vi "Find Largest Networks.vi"(8 "error in (no error)":errorcluster, 11 "Proto in":refnum<class "NetAn.lvclass">) -> (0 "error out":errorcluster, 2 "set":set{string}(c389), 3 "Proto out":refnum<class "NetAn.lvclass">)   [LabVIEW 2020, in "NetAn.lvclass"]
uses:
  NetAn.lvclass
  NetAn.lvclass/NetAn.ctl
panel:
  out "Numeric":i32
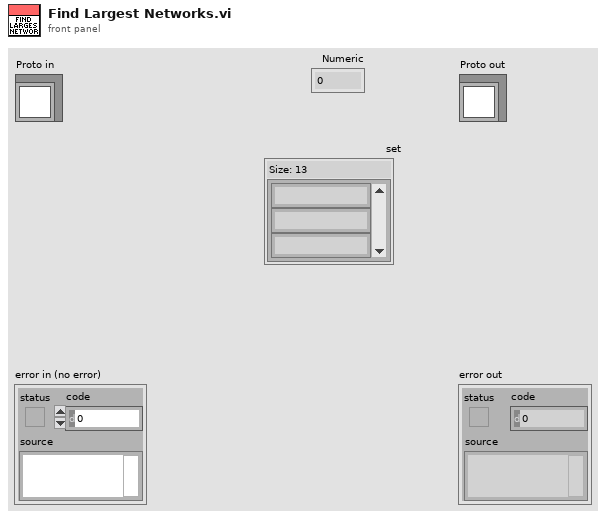
[diagram p1: front panel]
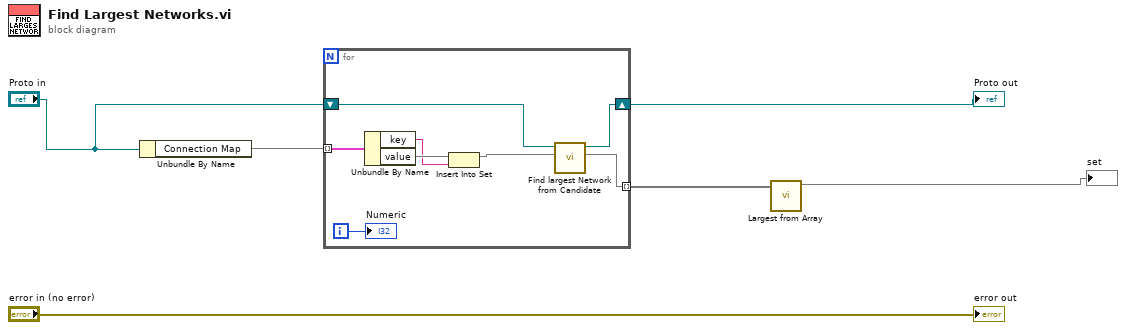
[diagram p0: block diagram]
diagram:
  n1 = Unbundle By Name("Proto in") -> ("Connection Map"=w5:map{string, set{string}})
  n2 = for {
    tunnel: w5 -> [w14] mode=indexing
    shift-right: [w8] -> w3
    shift-left: "Proto in" -> [w11]
    tunnel: [w9] -> w2 mode=indexing
    i -> [w7]
    n3 = Unbundle By Name(w14) -> ("key"=w12:string, "value"=w13:set{string})
    n4 = Insert Into Set(10:w12, 11:w13) -> (3:w10:set{string})  [unwired: 1 out]
    n5 = call "Find largest Network from Candidate.vi"("Candidate Network"=w10, "NetAn in"=w11) -> ("Largest Network"=w9:set{string}, "NetAn out"=w8:refnum<class "NetAn.lvclass">)  [unwired: 8 in]
    "Numeric" <- w7
  }
  "Proto out" <- w3
  n6 = call "Largest from Array.vi"("Array"=w2) -> ("Largest Network"=→"set":set{string})  [unwired: 10 in]
  "error out" <- "error in (no error)"
